vi "Ping.vi"(8 "error in (no error)":errorcluster, 11 "Sift Client in":refnum<class "Sift Client.lvclass">) -> (0 "error out":errorcluster, 2 "response":string, 3 "Sift Client out":refnum<class "Sift Client.lvclass">)   [LabVIEW 2024, in "Sift Client.lvlib" / "Sift Client.lvclass"]
doc: "Ping Sift.\n\nCall this VI to test that you can authenticate properly with Sift."
uses:
  Sift Client.lvclass
  Sift Client.lvclass/Sift Client.ctl
  <vilib>/addons/_JKI.lib/Serialization/JSON/JKI JSON Serialization.lvlib
  <vilib>/addons/_JKI.lib/REST Client/classes/REST Client/REST Client.lvclass
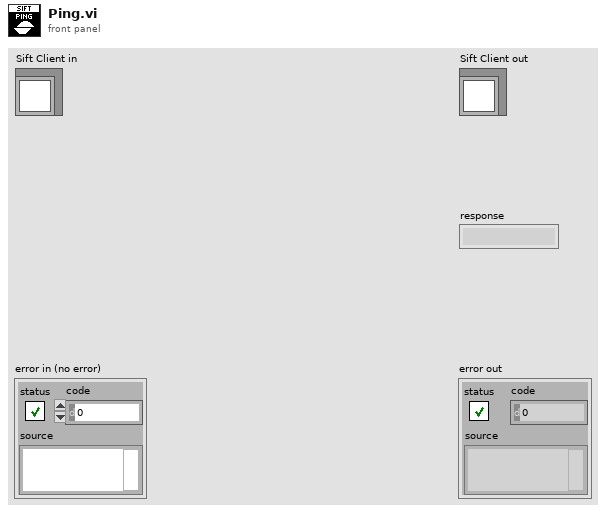
[diagram p1: front panel]
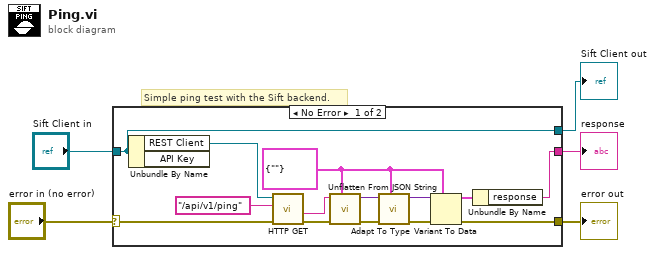
[diagram p0: block diagram]
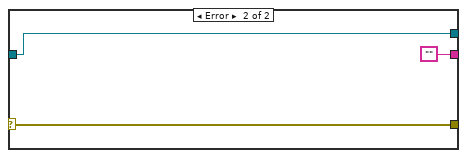
[diagram p2: hidden frame]
diagram:
  # "Simple ping test with the Sift backend."
  n1 = case shown="No Error" "error in (no error)" {
    selector: "error in (no error)" -> [w16 w22]
    tunnel: [w6 w22] -> w4
    tunnel: [w19 w21] -> w2
    tunnel: "Sift Client in" -> [w19 w21]
    tunnel: [w8 ""] -> w1
    frame No Error {
      w7 = cluster{"response":string} {"response"=""}
      n2 = Unbundle By Name(w19) -> ("REST Client"=w18:refnum<class "REST Client.lvclass">)  [unwired: 1 out]
      n3 = call-dynamic "HTTP GET.vi"("error in (no error)"=w16, "Path"="/api/v1/ping", "REST Client in"=w18) -> ("error out"=w15:errorcluster, "Response body"=w14:string)  [unwired: 3 in, 4 out]
      n4 = call <vilib>:"Unflatten From JSON String.vi"("Type and Defaults"=w7, "error in"=w15, "JSON String"=w14) -> ("error out"=w12:errorcluster, "Variant"=w13:variant)  [unwired: 7 in]
      n5 = call <vilib>:"Adapt To Type.vi"("Type and Defaults"=w7, "error in"=w12, "Variant in"=w13) -> ("error out"=w10:errorcluster, "Variant out"=w11:variant)  [unwired: 7 in]
      n6 = Variant To Data(error in=w10, type=w7, Variant=w11) -> (data=w9:cluster{"response":string}, error out=w6:errorcluster)
      n7 = Unbundle By Name(w9) -> ("response"=w8:string)
    }
    frame Error {
    }
  }
  "error out" <- w4
  "Sift Client out" <- w2
  "response" <- w1
